vi "Set Debugging.vi"(8 "error in (no error)":errorcluster, 10 "Debugging Control":bool, 11 "ProjectItem in":refnum<vi>) -> (0 "error out":errorcluster)   [LabVIEW 2018]
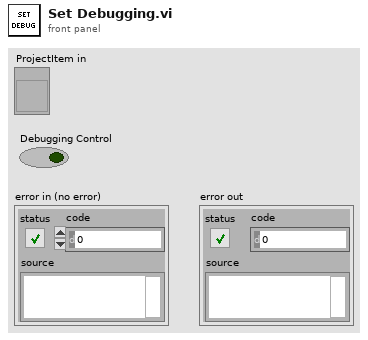
[diagram p1: front panel]
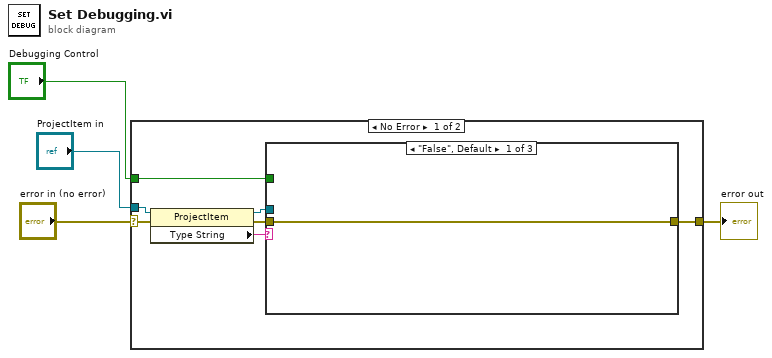
[diagram p0: block diagram]
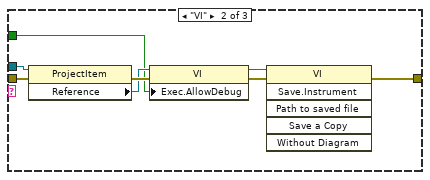
[diagram p2: hidden frame]
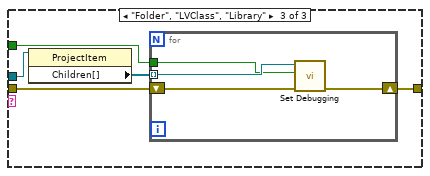
[diagram p3: hidden frame]
diagram:
  n1 = case shown="No Error" "error in (no error)" {
    selector: "error in (no error)" -> [w6 w30]
    tunnel: "ProjectItem in" -> [w11 _]
    tunnel: "Debugging Control" -> [w8 _]
    tunnel: [w7 w30] -> w3
    frame No Error {
      n2 = property class="ProjectItem"(reference=w11, error in=w6) -> (reference out=w9:refnum<vi>, error out=w10:errorcluster, "Type String"=w5:string)
      n3 = case shown="\"False\", Default" w5 {
        tunnel: w10 -> [w12 w15 w22]
        tunnel: w9 -> [_ w16 w25]
        tunnel: w8 -> [_ w13 w23]
        tunnel: [w12 w18 w21] -> w7
        frame "False", Default {
        }
        frame "VI" {
          n4 = property class="ProjectItem"(reference=w16, error in=w15) -> (error out=w17:errorcluster, "Reference"=w14:refnum<vi>)  [unwired: 1 out]
          n5 = property class="VI"(reference=w14, error in=w17, "Exec.AllowDebug"=w13) -> (reference out=w20:refnum<vi>, error out=w19:errorcluster)
          n6 = invoke class="VI" method="Save.Instrument"(reference=w20, error in=w19) -> (error out=w18:errorcluster)  [unwired: 4 in, 5 out]
        }
        frame "Folder", "LVClass", "Library" {
          n7 = property class="ProjectItem"(reference=w25) -> ("Children[]"=w24:refnum<vi>[])  [unwired: 1 in, 2 out]
          n8 = for {
            tunnel: w24 -> [w29] mode=indexing
            tunnel: w23 -> [w28]
            shift-right: [w26] -> w21
            shift-left: w22 -> [w27]
            n9 = call "Set Debugging.vi"("error in (no error)"=w27, "Debugging Control"=w28, "ProjectItem in"=w29) -> ("error out"=w26:errorcluster)  [unwired: 8 in]
          }
        }
      }
    }
    frame Error {
    }
  }
  "error out" <- w3
